vi "例4.2 测试程序的运行时间.vi"() -> ()   [LabVIEW 2017]
panel:
  out "时间":u32
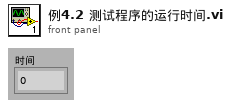
[diagram p1: front panel]
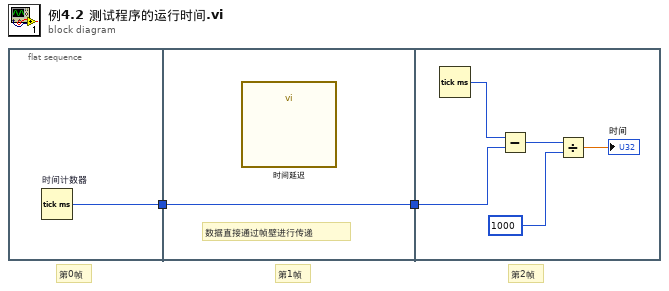
[diagram p0: block diagram]
diagram:
  # "第2帧"
  # "第1帧"
  # "第0帧"
  n1 = flat-sequence {
    tunnel: [w3] -> w2
    tunnel: w2 -> [w4]
    tunnel: [w4] -> w1
    tunnel: w1 -> [w8]
    frame #0 {
      n2 = Tick Count (ms) "时间计数器"() -> (millisecond timer value=w3:u32)
    }
    frame #1 {
      # "数据直接通过帧壁进行传递"
      n3 = call "时间延迟"() -> ()  [unwired: 11 in, 1 out]
    }
    frame #2 {
      n4 = Tick Count (ms)() -> (millisecond timer value=w9:u32)
      n5 = Subtract(x=w9, y=w8) -> (x-y=w7:u32)
      n6 = Divide(x=w7, y=u32 1000) -> (x/y=→"时间":dbl)
    }
  }
